vi "Start Process.vi"(8 "error in (no error)":errorcluster, 11 "CoolAppProcess in":refnum<class "CoolAppProcess.lvclass">) -> (0 "error out":errorcluster, 3 "CoolAppProcess out":refnum<class "CoolAppProcess.lvclass">)   [LabVIEW 2020, in "LAF2024Q2.lvlib" / "CoolAppProcess.lvclass"]
uses:
  CoolAppProcess.lvclass
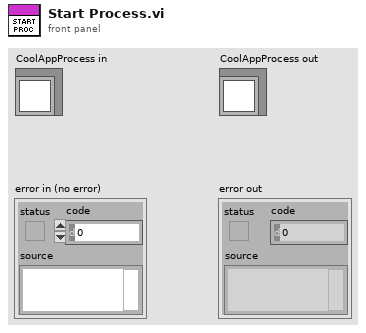
[diagram p1: front panel]
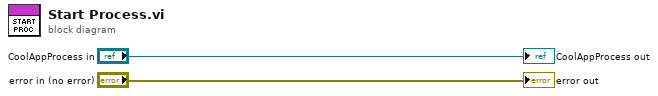
[diagram p0: block diagram]
diagram:
  "error out" <- "error in (no error)"
  "CoolAppProcess out" <- "CoolAppProcess in"
